vi "MeasureCommand.vi"(11 "Port":enum8{"ONE", "TWO"}(ring)) -> (3 "ByteArrayToSend":u8[](array[numeric]) format="%x")   [LabVIEW 2019]
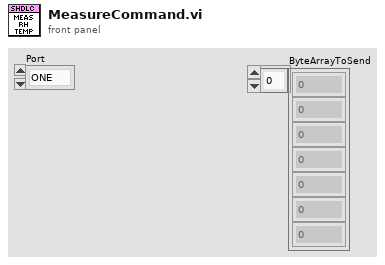
[diagram p1: front panel]
types:
  T1 = cluster{"Port":u8, "I2CAdress":u8, "RX Length":u32, "Timeout":u32, "TX Data":u8[]}
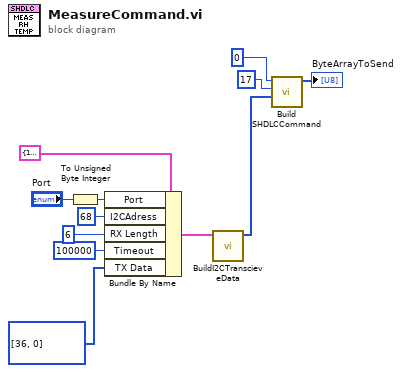
[diagram p0: block diagram]
diagram:
  n1 = To Unsigned Byte Integer(number="Port") -> (unsigned 8bit integer=w1:u8)
  n2 = Bundle By Name(cluster=T1 {"Port"=1, "I2CAdress"=1, "RX Length"=1, "Timeout"=1, "TX Data"=[]} ("Cluster"), "Port"=w1, "I2CAdress"=u8 68, "RX Length"=u32 6, "Timeout"=u32 100000, "TX Data"=u8[] [36, 0]) -> (w9:T1)
  n3 = call "BuildI2CTranscieveData.vi"("Cluster"=w9) -> ("I2CDataAsByteArray"=w2:u8[])  [unwired: 9 in, 1 out]
  n4 = call "Build SHDLCCommand.vi"("Data"=w2, "CommandID"=u8 17, "SlaveAdress"=u8 0) -> ("ByteArrayToSend"=→"ByteArrayToSend":u8[])  [unwired: 8 in]
